vi "ET2604 - Read Temperature.vi"(7 "error in (no error)":errorcluster, 10 "VISA resource name":refnum<visa-resource-name>) -> (0 "error out":errorcluster, 2 "Data":sgl, 3 "VISA resource name out":refnum<visa-resource-name>)   [LabVIEW 2017]
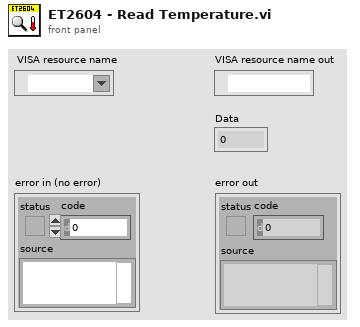
[diagram p1: front panel]
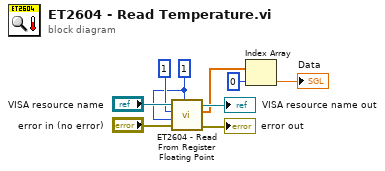
[diagram p0: block diagram]
diagram:
  w4 = u16 1 ("Num Of Reg (1)")
  n1 = call "ET2604 - Read From Register Floating Point.vi"("Num Of Reg (1)"=w4, "error in (no error)"="error in (no error)", "Register Address (0)"=w4, "Unit Address (1)"=u8 1, "VISA session"="VISA resource name") -> ("error out"=→"error out":errorcluster, "Data"=w2:sgl[], "dup VISA session"=→"VISA resource name out":refnum<visa-resource-name>)  [unwired: 4 in]
  n2 = Index Array(array=w2, index=0) -> (element=→"Data":sgl)
